vi "Write Raw CMD - Multiple Devices.vi"(0 "Data Out":string, 11 "error in":errorcluster, 12 "Log (T)":bool=TRUE, 13 "Dev Mask (All)":bool[](array[boolean])=[TRUE, TRUE, TRUE, TRUE, TRUE, TRUE], 14 "FPGA":T1) -> (15 "error out":errorcluster)   [LabVIEW 2017, in "Host SRL.lvlib"]
uses:
  Host SRL.lvlib
  Type Defs/WSVCAP SHL FPGA Enum.ctl
panel:
  out "Socket Mask":u32=1 format="%06x"
  out "Data Out":u8[][](array[numeric]) format="%02x"
  # "Dev 01"
  # "Dev 02"
  # "Dev 03"
  # "Dev 04"
  # "Dev 05"
  # "Dev 06"
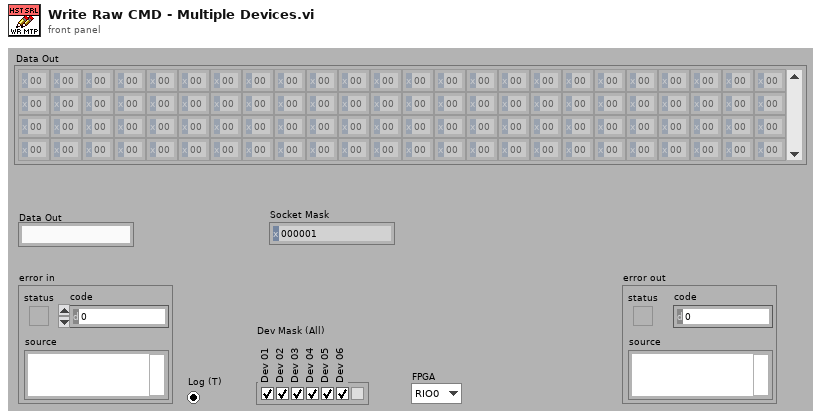
[diagram p1: front panel]
types:
  T1 = typedef "WSVCAP SHL FPGA Enum.ctl" = enum16{"RIO0", "RIO1"}
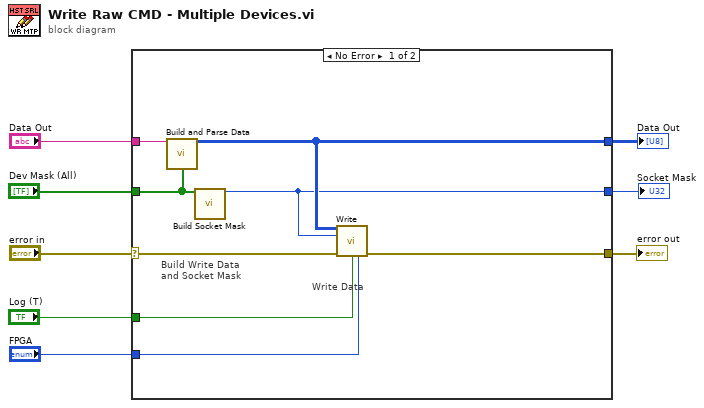
[diagram p0: block diagram]
diagram:
  n1 = case shown="No Error" "error in" {
    selector: "error in" -> [w16 _]
    tunnel: [w15 _] -> w8
    tunnel: "Data Out" -> [w14 _]
    tunnel: [w13 _] -> w5
    tunnel: [w9 _] -> w4
    tunnel: "Log (T)" -> [w12 _]
    tunnel: "FPGA" -> [w11 _]
    tunnel: "Dev Mask (All)" -> [w10 _]
    frame No Error {
      # "Write Data"
      # "Build Write Data and Socket Mask"
      n2 = call "Build and Parse Data.vi"("SRL Message Out"=w14, "Dev Mask (All)"=w10) -> ("SRL Data Out [U8]"=w13:u8[][])  [unwired: 12 in, 1 out]
      n3 = call "Build Socket Mask.vi"("Dev Mask (All)"=w10) -> ("Socket Mask [U32]"=w9:u32)  [unwired: 14 in]
      n4 = call "Write.vi"("SRL Data Out"=w13, "Socket Mask"=w9, "error in"=w16, "Log (T)"=w12, "FPGA"=w11) -> ("error out"=w15:errorcluster)  [unwired: 10 in]
    }
    frame Error {
    }
  }
  "error out" <- w8
  "Data Out" <- w5
  "Socket Mask" <- w4
